vi "Object Storage Without Type Preservation.vi"(8 "error in (no error)":errorcluster, 10 "Action":u16(ring) items=["Store Object", "Retrieve Object"], 11 "Object in":refnum<class "Parent.lvclass">) -> (0 "error out":errorcluster, 3 "Object out":refnum<class "Parent.lvclass">)   [LabVIEW 2023, in "Parent.lvclass"]
doc: "This VI does not preserve the run-time type of the object passed in to the object passed out."
uses:
  Parent.lvclass
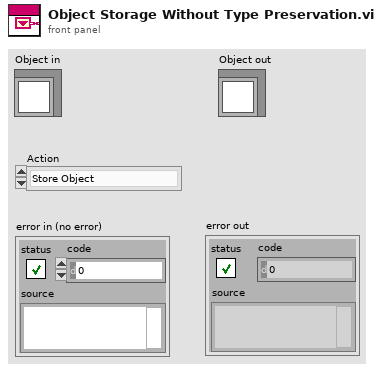
[diagram p1: front panel]
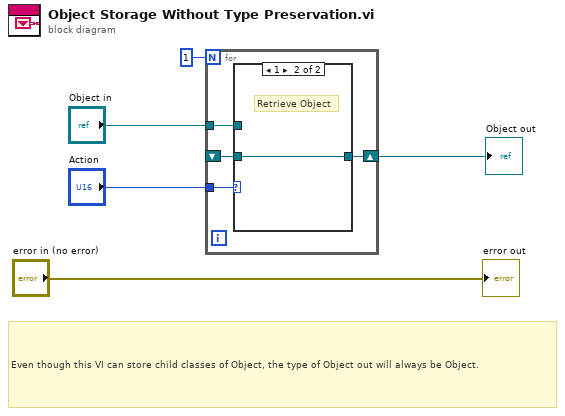
[diagram p0: block diagram]
diagram:
  # "Even though this VI can store child classes of Object, the type of Object out will always be Object."
  n1 = for {
    N: 1 -> [_]
    shift-right: [w8] -> w4
    shift-left: _ -> [w6]
    tunnel: "Action" -> [w9]
    tunnel: "Object in" -> [w7]
    n2 = case shown="1" w9 {
      tunnel: [w10 w11] -> w8
      tunnel: w7 -> [w10 _]
      tunnel: w6 -> [_ w11]
      frame 0, Default {
        # "Store Object"
      }
      frame 1 {
        # "Retrieve Object"
      }
    }
  }
  "Object out" <- w4
  "error out" <- "error in (no error)"
